vi "pxie_7962_fpga.vi"() -> ()   [LabVIEW 2014]
uses:
  <instrlib>/_niInstr/Streaming/v1/Common/Stream State.ctl
  FPGA_Controls/Init.ctl
  <vilib>/Platform/TimedLoop/XDataNode/timing_clust.ctl
  <vilib>/Platform/TimedLoop/XDataNode/nitl_modes.ctl
  <vilib>/Platform/TimedLoop/XDataNode/wakeup.ctl
  FPGA_Controls/Acquisition FIFOs Cluster.ctl
  <vilib>/rvi/Emulation/niFpgaSctlEmulationGetInTimedLoop.vi
  <vilib>/rvi/Emulation/niFpgaEmulationReportErrorSimple.vi
  <vilib>/rvi/Emulation/niFpgaGetClockAttributes.vi
  <vilib>/rvi/Emulation/niFpgaCriticalErrorInLSC.vi
  <vilib>/rvi/eio/common/nirviEmuTemplateMethod_errors.vi
  <instrlib>/_niInstr/Basic Elements/v1/FPGA/Private/Count Up U32.vi
  <vilib>/rvi/Memory/Memory_Emulation/niFpgaMemoryFastEmulationDramWriteAndRequestData.vi
  <vilib>/rvi/Memory/Memory_Emulation/niFpgaMemoryEmulationDramWriteAndRequestData.vi
  <vilib>/rvi/DataTransferAndStorage/Container/Common/niFpgaContainerGetUniqueNameForEmu.vi
  <vilib>/rvi/Memory/Memory_Emulation/niFpgaMemoryEmulationDramWriteAndRequestDataApplyByteEnables.vi
  <vilib>/rvi/interface/RandomDataEmulation/niFpgaRandomDataHandleErrors.vi
  <instrlib>/_niInstr/Basic Elements/v1/FPGA/Private/Count Up U64.vi
  <vilib>/rvi/DataTransferAndStorage/Container/Common/niFpgaContainerExecOnDevCompGetState.vi
  <vilib>/rvi/Emulation/niFpgaEmulationIsFPGAContextNoSignature.vi
  <vilib>/rvi/errors/niFpgaSetErrorForExecOnDevCompSimple.vi
  <vilib>/rvi/eio/common/nirviEmuReportErrorAndStop.vi
  <vilib>/rvi/FIFO/Fifo_Resource/nirvififoEmulationSetSize.vi
  <vilib>/rvi/FIFO/Fifo_Resource/nirviFifoEmulationQueueMgr.vi
  <instcachedir>/0/nirviFifoEmulationQueueMgr_E5CAEC123FF24DC58D834DCA3CDAA9B5.lvgen/nirviFifoEmulationQueueMgr_E5CAEC123FF24DC58D834DCA3CDAA9B5_003.vi
  <vilib>/rvi/FIFO/Fifo_Resource/nirvififoEmulationDetermineInputValidOut.vi
  <vilib>/rvi/FIFO/Fifo_Resource/nirvififoEmulationCreateLock.vi
  <vilib>/rvi/Emulation/niFpgaProcessEmulError.vi
  <vilib>/rvi/FIFO/Fifo_Resource/nirvififoEmulationObtainLock.vi
  <vilib>/rvi/FIFO/Fifo_Resource/nirvififoEmulationReleaseLock.vi
  <vilib>/rvi/occurrence/nirviWaitOnOccurrenceBase.vi
  <vilib>/rvi/errors/nirviReportUnexpectedCaseInternalError.vi
  <vilib>/rvi/errors/nirviReportUnexpectedCaseInternalError (U32).vi
  <vilib>/Utility/error.llb/Clear Errors.vi
  <vilib>/Platform/TimedLoop/XDataNode/XDataNode.xnode
  <vilib>/eio/EIONode/EIONode.xnode
  <vilib>/rvi/DataTransferAndStorage/Container/XNode/niFpgaContainer.xnode
  <vilib>/rvi/Memory/Memory_Emulation/niFpgaMemoryEmulationDramRetrieveData.vi
  <vilib>/rvi/interface/RandomDataEmulation/nirviRandomDataFpgaReadWriteTemplate.vi
  <vilib>/rvi/FIFO/Fifo_Resource/niFpgaFifoEmulationRefIn.vi
  <vilib>/Platform/TimedLoop/XDataNode/XDNodeRunTimeDep.lvlib
  <instrlib>/_niInstr/Streaming/v1/FPGA/niInstr Streaming v1 FPGA.lvlib
  <instrlib>/_niInstr/Basic Elements/v1/FPGA/niInstr Basic Elements v1 FPGA.lvlib
  <instrlib>/_niInstr/Streaming/v1/Common/niInstr Streaming v1 Common.lvlib
panel:
  in  "manual\ntrigger":bool
  out "Writes to DRAM":u64
  out "DRAM Write address":u32
  in  "Reset DRAM write address":bool
  in  "Reset DRAM read address":bool
  in  "trigger \ndelay":u64
  in  "Clear Trigger":bool
  in  "Output Debug Data":bool
  out "stream.metadata 0":u64
  in  "stream.request state 0":T1
  out "stream.samples transferred 0":u64
  out "stream.state 0":T1
  in  "stream.num samples 0":u64
  out "Writes to DMA":u64
  out "Samples Aquired":u64
  out "IO Module Init Done":bool
  in  "stream.num samples 1":u64
  out "stream.state 1":T1
  out "stream.samples transferred 1":u64
  in  "stream.request state 1":T1
  out "stream.metadata 1":u64
  # "Stream 0 (Aquisition Stream)"
  # "Throughput Diagnostics"
  # "Stream 1 (Transfer to Host Stream)"
  # "Settings & Resets"
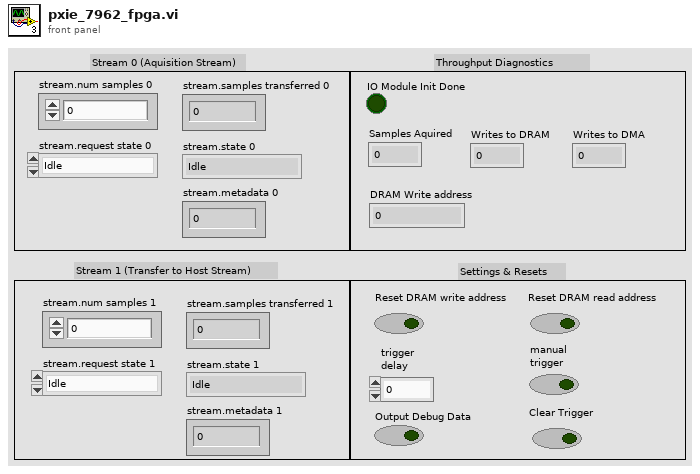
[diagram p1: front panel]
types:
  T1 = typedef "niInstr Streaming v1 Common.lvlib/Stream State.ctl" = enum8{"Idle", "Finite Transfer", "Continuous", "Done", "Error", "Not Ready", "Cancel"}
  T2 = typedef "Init.ctl" = enum16{"InitIOCheck", "ADCConfigForWrite", "SPIConfigWaitForSPIIdleFalse", "SPIConfigWaitForSPIIdleTrue", "ADCTurnOffInternalHighPassFilter", "SPIHighPassWaitForSPIIdleFalse", "SPIHighPassWaitForSPIIdleTrue"}
  T3 = typedef "XDNodeRunTimeDep.lvlib/timing_clust.ctl" = cluster{"Expected End [f-1]":u64, "Actual End [f-1]":u64, "Finished Late? [f-1]":bool, "Expected End [i-1]":u64, "Actual End [i-1]":u64, "Finished Late? [i-1]":bool, "Expected Start [i]":u64, "Actual Start [i]":u64, "Expected Start [f]":u64, "Actual Start [f]":u64, "Source Name":string, "Structure Name":string, "Period":i64, "Deadline":i64, "Offset":i64, "Start":i64, "Priority":i32, "Timeout":i32, "Mode":T4, "Wakeup Reason":T5, "Error":errorcluster, "Source Type":string, "Secondary Source Type":string, "Global End Time":u64, "Global Start Time":u64, "Frame Duration":u64, "Iteration Duration":u64, "Assigned CPU":i32, "I/O Scan Engine Mode":u32}
  T4 = typedef "XDNodeRunTimeDep.lvlib/nitl_modes.ctl" = enum32{"No Change", "Process missed periods, maintain original phase", "Discard missed periods, maintain original phase", "Process missed periods, ignore original phase", "Discard missed periods, ignore original phase"}
  T5 = typedef "XDNodeRunTimeDep.lvlib/wakeup.ctl" = enum32{"Normal", "Aborted", "Asynchronous wakeup", "Timing source error", "Timed loop error", "Timeout"}
  T6 = typedef "Acquisition FIFOs Cluster.ctl" = cluster{"FIFO 0":refnum<k21>, "FIFO 1":refnum<k21>, "FIFO 2":refnum<k21>, "FIFO 3":refnum<k21>, "FIFO 4":refnum<k21>, "FIFO 5":refnum<k21>, "FIFO 6":refnum<k21>, "FIFO 7":refnum<k21>}
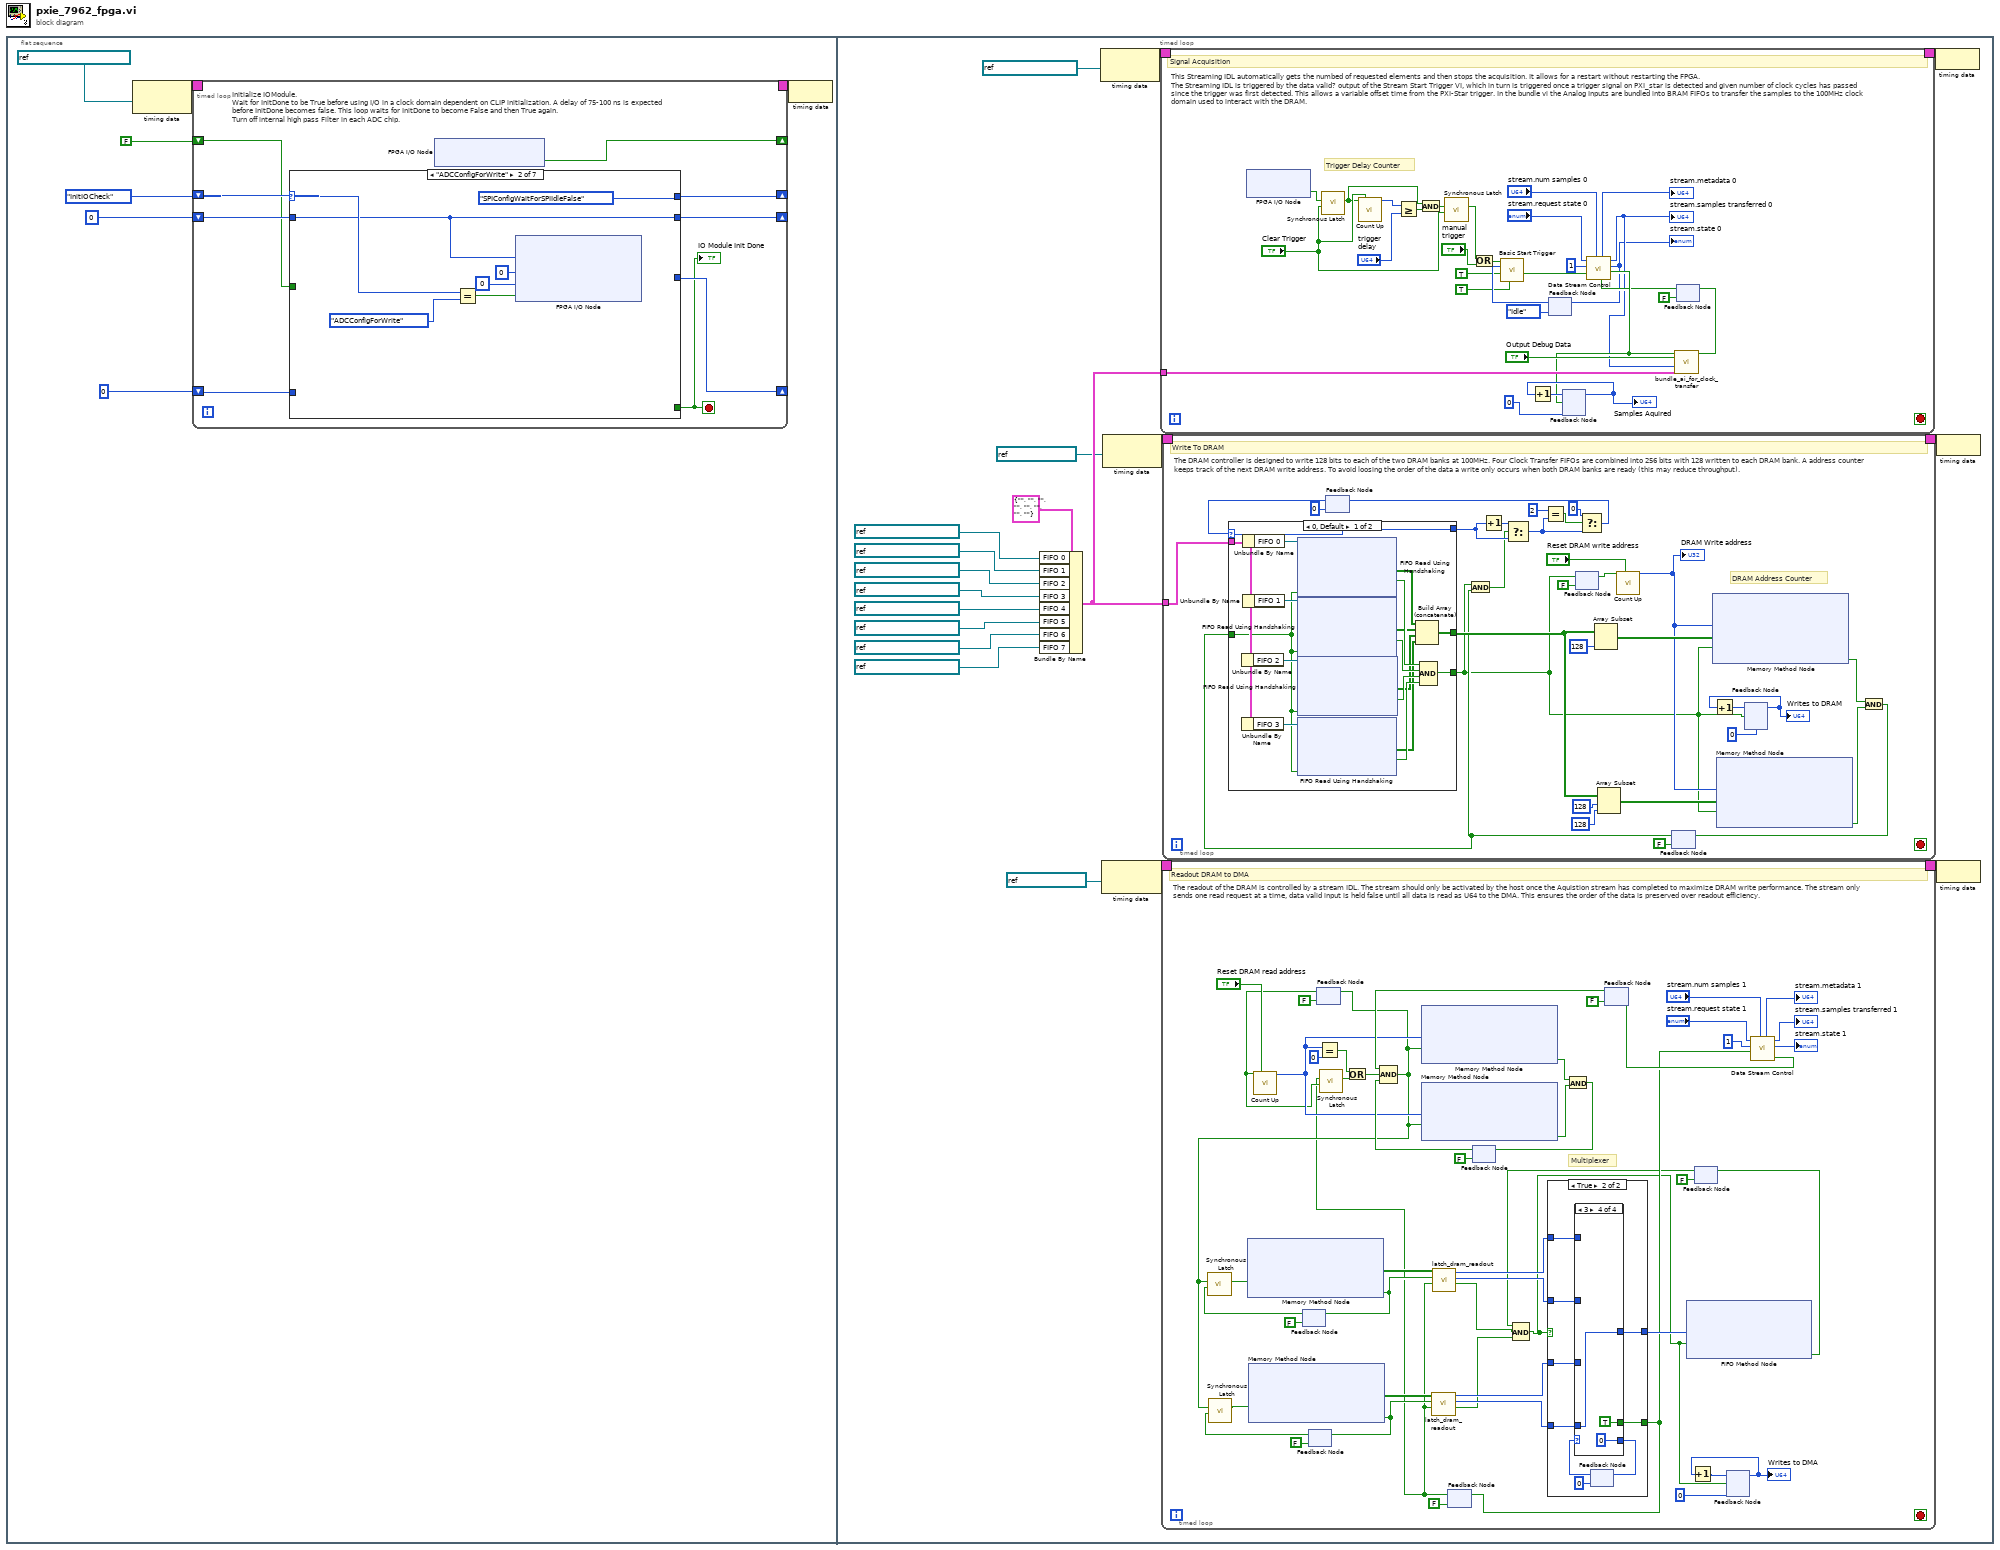
[diagram p0: block diagram]
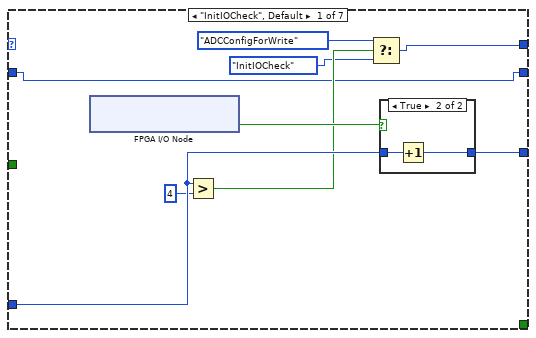
[diagram p2: hidden frame]
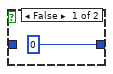
[diagram p3: hidden frame]
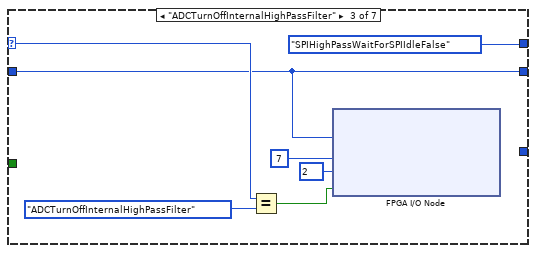
[diagram p4: hidden frame]
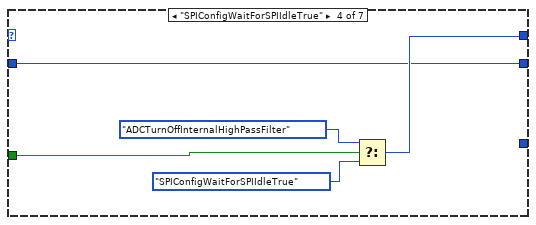
[diagram p5: hidden frame]
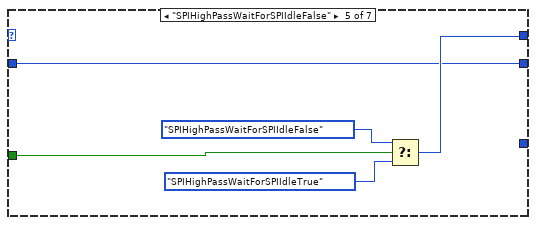
[diagram p6: hidden frame]
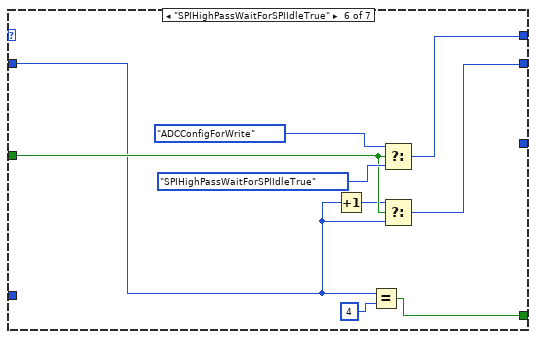
[diagram p7: hidden frame]
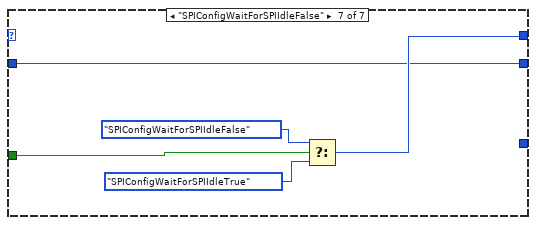
[diagram p8: hidden frame]
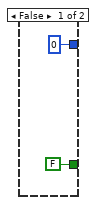
[diagram p9: hidden frame]
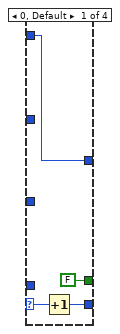
[diagram p10: hidden frame]
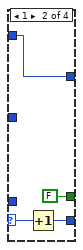
[diagram p11: hidden frame]
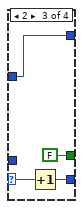
[diagram p12: hidden frame]
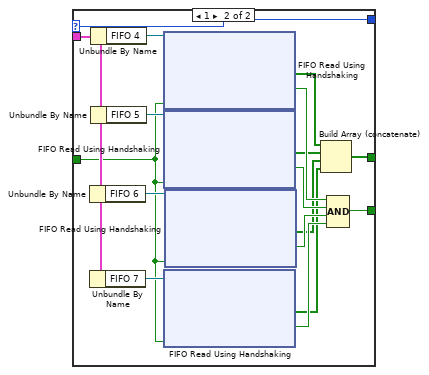
[diagram p13: hidden frame]
diagram:
  n1 = flat-sequence {
    frame #0 {
      # "Initialize IOModule.\nWait for InitDone to be True before using I/O in a clock domain dependent on CLIP initialization. A delay of 75-100 ns is expected before InitDone becomes false. This loop waits for InitDone to become False and then True again.\nTurn off internal high pass Filter in each ADC chip."
      n2 = node-c288(refnum<k21> "40 MHz Onboard Clock" ("Source Name")) -> (w7:T3)
      n3 = timed-loop {
        shift-right: [w16] -> _
        shift-left: u16 0 -> [w15]
        timing: w7 -> [_]
        timing-out: [_] -> w6
        shift-right: [w14] -> _
        shift-left: Init."InitIOCheck" -> [w13]
        shift-right: [w11] -> _
        shift-left: u8 0 -> [w12]
        shift-right: [w10] -> _
        shift-left: FALSE ("IO Module\\cSpiIdle") -> [w9]
        stop <- w8 stop-if-true
        n4 = case shown="\"ADCConfigForWrite\"" w13 {
          selector: w13 -> [_ w32 w39 _ _ _ _]
          tunnel: [w25 _ _ _ _ _ _] -> w16
          tunnel: w15 -> [w24 _ _ _ _ _ _]
          tunnel: [w21 Init."SPIConfigWaitForSPIIdleFalse" Init."SPIHighPassWaitForSPIIdleFalse" ("y") w44 w50 w59 w63] -> w14
          tunnel: [_ _ _ _ _ w57 _] -> w8
          tunnel: w12 -> [w17 w30 w37 w43 w48 w54 w62]
          tunnel: [w17 w30 w37 w43 w48 w53 w62] -> w11
          tunnel: w9 -> [_ _ _ w45 w49 w56 w66]
          frame "InitIOCheck", Default {
            n5 = xnode "FPGA I/O Node"() -> ("IO Module\\InitDone"=w22:bool)  [unwired: 1 in, 1 out]
            n6 = Greater?(x=w24, y=u16 4) -> (0:w20:bool)
            n7 = Select(t=Init."ADCConfigForWrite", s=w20, f=Init."InitIOCheck") -> (s? t:f=w21:T2)
            n8 = case shown="True" w22 {
              tunnel: [u16 0 w28] -> w25
              tunnel: w24 -> [_ w27]
              frame False {
              }
              frame True {
                n9 = Increment(x=w27) -> (x+1=w28:u16)
              }
            }
          }
          frame "ADCConfigForWrite" {
            n10 = Equal?(x=w32, y=Init."ADCConfigForWrite") -> (x = y?=w33:bool)
            n11 = xnode "FPGA I/O Node"("IO Module\\cSpiDevice"=w30, "IO Module\\cSpiAddr"=u16 0 ("IO Module\\cSpiAddr"), "IO Module\\cSpiWrData"=u16 0 ("IO Module\\cSpiWrData"), "IO Module\\cSpiWriteEn"=w33) -> ()  [unwired: 4 in, 4 out]
          }
          frame "ADCTurnOffInternalHighPassFilter" {
            n12 = Equal?(x=w39, y=Init."ADCTurnOffInternalHighPassFilter") -> (x = y?=w40:bool)
            n13 = xnode "FPGA I/O Node"("IO Module\\cSpiDevice"=w37, "IO Module\\cSpiAddr"=u16 7 ("IO Module\\cSpiAddr"), "IO Module\\cSpiWrData"=u16 2 ("IO Module\\cSpiWrData"), "IO Module\\cSpiWriteEn"=w40) -> ()  [unwired: 4 in, 4 out]
          }
          frame "SPIConfigWaitForSPIIdleTrue" {
            n14 = Select(t=Init."ADCTurnOffInternalHighPassFilter", s=w45, f=Init."SPIConfigWaitForSPIIdleTrue") -> (s? t:f=w44:T2)
          }
          frame "SPIHighPassWaitForSPIIdleFalse" {
            n15 = Select(t=Init."SPIHighPassWaitForSPIIdleFalse", s=w49, f=Init."SPIHighPassWaitForSPIIdleTrue") -> (s? t:f=w50:T2)
          }
          frame "SPIHighPassWaitForSPIIdleTrue" {
            n16 = Increment(x=w54) -> (x+1=w55:u8)
            n17 = Equal?(x=w54, y=u8 4) -> (x = y?=w57:bool)
            n18 = Select(t=Init."ADCConfigForWrite", s=w56, f=Init."SPIHighPassWaitForSPIIdleTrue") -> (s? t:f=w59:T2)
            n19 = Select(t=w55, s=w56, f=w54) -> (s? t:f=w53:u8)
          }
          frame "SPIConfigWaitForSPIIdleFalse" {
            n20 = Select(t=Init."SPIConfigWaitForSPIIdleFalse", s=w66, f=Init."SPIConfigWaitForSPIIdleTrue") -> (s? t:f=w63:T2)
          }
        }
        "IO Module Init Done" <- w8
        n21 = xnode "FPGA I/O Node"() -> ("IO Module\\cSpiIdle"=w10:bool)  [unwired: 1 in, 1 out]
      }
      n22 = node-c288(w6) -> ()
    }
    frame #1 {
      n23 = Bundle By Name(cluster=T6 {"FIFO 0"="", "FIFO 1"="", "FIFO 2"="", "FIFO 3"="", "FIFO 4"="", "FIFO 5"="", "FIFO 6"="", "FIFO 7"=""} ("FIFO Refs"), "FIFO 0"=refnum<k21> "Clock Transfer FIFO 0" ("FIFO In"), "FIFO 1"=refnum<k21> "Clock Transfer FIFO 1" ("FIFO In"), "FIFO 2"=refnum<k21> "Clock Transfer FIFO 2" ("FIFO In"), "FIFO 3"=refnum<k21> "Clock Transfer FIFO 3" ("FIFO In"), "FIFO 4"=refnum<k21> "Clock Transfer FIFO 4" ("FIFO In"), "FIFO 5"=refnum<k21> "Clock Transfer FIFO 5" ("FIFO In"), "FIFO 6"=refnum<k21> "Clock Transfer FIFO 6" ("FIFO In"), "FIFO 7"=refnum<k21> "Clock Transfer FIFO 7" ("FIFO In")) -> (w76:T6)
      n24 = node-c288(refnum<k21> "IO Module Clock 0" ("Source Name")) -> (w91:T3)
      n25 = node-c288(refnum<k21> "100 MHz Clock" ("Source Name")) -> (w87:T3)
      n26 = node-c288(refnum<k21> "100 MHz Clock" ("Source Name")) -> (w89:T3)
      n27 = timed-loop {
        timing: w91 -> [_]
        timing-out: [_] -> w90
        tunnel: w76 -> [w268]
        stop <- _ stop-if-true
        # "Trigger Delay Counter"
        # "This Streaming IDL automatically gets the numbed of requested elements and then stops the acquisition. It allows for a restart without restarting the FPGA. \nThe Streaming IDL is triggered by the data valid? output of the Stream Start Trigger VI, which in turn is triggered once a trigger signal on PXI_star is detected and given number of clock cycles has passed since the trigger was first detected. This allows a variable offset time from the PXI-Star trigger. In the bundle vi the Analog Inputs are bundled into BRAM FIFOs to transfer the samples to the 100MHz clock domain used to interact with the DRAM."
        # "Signal Acquisition"
        n28 = xnode "FPGA I/O Node"() -> ("PXI_Star"=w254:bool)  [unwired: 1 in, 1 out]
        n29 = call <instrlib>:"Synchronous Latch.vi"("clear"="Clear Trigger", "set"=w254) -> ("out"=w248:bool)  [unwired: 9 in]
        n30 = call-poly <instrlib>:"Count Up.vi"("increment"=w248, "reset"="Clear Trigger") -> ("count out"=w253:u64)  [unwired: 13 in]
        n31 = Greater Or Equal?(x=w253, y="trigger \ndelay") -> (x >= y?=w249:bool)
        n32 = And(x=w248, y=w249) -> (x .and. y?=w247:bool)
        n33 = call <instrlib>:"Synchronous Latch.vi"("clear"="Clear Trigger", "set"=w247) -> ("out"=w246:bool)  [unwired: 9 in]
        n34 = Or(x=w246, y="manual\ntrigger") -> (x .or. y?=w244:bool)
        n35 = feedback #1(Stream_State."Idle" ("stream.state 0")) -> (w258:T1)
        n36 = call <instrlib>:"Basic Start Trigger.vi"("ready for start trigger"=TRUE, "data valid?"=TRUE, "stream.state"=w258, "start trigger"=w244) -> ("data valid"=w251:bool)  [unwired: 7 in]
        n37 = feedback #2(u64 0) -> (w269:u64)
        "Samples Aquired" <- w269
        n38 = Increment(x=w269) -> (x+1=w270:u64)
        n39 = feedback #3(FALSE ("Ready for Input")) -> (w265:bool)
        n40 = call <instrlib>:"Data Stream Control.vi"("ready for input?"=w265, "stream.num samples 0"="stream.num samples 0", "data valid"=w251, "element count"=u16 1, "stream.request state 0"="stream.request state 0") -> ("send data"=w266:bool, "stream.state 0"=w262:T1, "stream.samples transferred 0"=w263:u64, "stream.metadata 0"=→"stream.metadata 0":u64)  [unwired: 2 in, 1 out]
        "stream.state 0" <- w262
        "stream.samples transferred 0" <- w263
        n41 = feedback-in #1(w262) -> ()
        n42 = feedback-in #2(w270, w266) -> ()
        n43 = call "bundle_ai_for_clock_transfer.vi"("FIFO Refs"=w268, "sample"=w263, "Debug"="Output Debug Data", "Input Valid"=w266) -> ("Ready for Input"=w273:bool)  [unwired: 7 in]
        n44 = feedback-in #3(w273) -> ()
      }
      n45 = timed-loop {
        timing: w87 -> [_]
        timing-out: [_] -> w86
        stop <- _ stop-if-true
        # "Multiplexer"
        # "The readout of the DRAM is controlled by a stream IDL. The stream should only be activated by the host once the Aquistion stream has completed to maximize DRAM write performance. The stream only sends one read request at a time, data valid input is held false until all data is read as U64 to the DMA. This ensures the order of the data is preserved over readout efficiency."
        # "Readout DRAM to DMA"
        n46 = feedback #4(FALSE ("Output Valid")) -> (w106:bool)
        n47 = feedback #5(FALSE ("Output Valid")) -> (w103:bool)
        n48 = feedback #6(FALSE) -> (w113:bool)
        n49 = call-poly <instrlib>:"Count Up.vi"("increment"=w113, "reset"="Reset DRAM read address") -> ("count out"=w118:u32)  [unwired: 13 in]
        n50 = Equal?(x=w118, y=u32 0) -> (x = y?=w115:bool)
        n51 = feedback #7(FALSE) -> (w99:bool)
        n52 = call <instrlib>:"Synchronous Latch.vi"("clear"=w113, "set"=w99) -> ("out"=w114:bool)  [unwired: 9 in]
        n53 = Or(x=w115, y=w114) -> (x .or. y?=w116:bool)
        n54 = feedback #8(FALSE) -> (w120:bool)
        n55 = feedback #9(FALSE ("request data")) -> (w119:bool)
        n56 = Compound Arithmetic op=AND(w119, w116, w120) -> (w102:bool)
        n57 = call <instrlib>:"Synchronous Latch.vi"("clear"=w106, "set"=w102) -> ("out"=w109:bool)  [unwired: 9 in]
        n58 = call <instrlib>:"Synchronous Latch.vi"("clear"=w103, "set"=w102) -> ("out"=w108:bool)  [unwired: 9 in]
        n59 = xnode ("Memory Method Node")("Ready for Output"=w109) -> ("Data"=w132:bool[], "Output Valid"=w107:bool)  [unwired: 1 in, 1 out]
        n60 = xnode ("Memory Method Node")("Ready for Output"=w108) -> ("Data"=w101:bool[], "Output Valid"=w100:bool)  [unwired: 1 in, 1 out]
        n61 = feedback-in #4(w107) -> ()
        n62 = feedback-in #5(w100) -> ()
        n63 = feedback-in #6(w102) -> ()
        n64 = xnode ("Memory Method Node")("Address"=w118, "Input Valid"=w102) -> ("Ready for Input"=w124:bool)  [unwired: 1 in, 1 out]
        n65 = xnode ("Memory Method Node")("Address"=w118, "Input Valid"=w102) -> ("Ready for Input"=w123:bool)  [unwired: 1 in, 1 out]
        n66 = call "latch_dram_readout.vi"("Reset"=w99, "Output Valid"=w100, "Data"=w101) -> ("Lateched Output Valid"=w92:bool, "latched U64 1"=w97:u64, "lateched U64 0"=w98:u64)  [unwired: 6 in]
        n67 = call "latch_dram_readout.vi"("Reset"=w99, "Output Valid"=w107, "Data"=w132) -> ("Lateched Output Valid"=w93:bool, "latched U64 1"=w131:u64, "lateched U64 0"=w130:u64)  [unwired: 6 in]
        n68 = And(x=w124, y=w123) -> (x .and. y?=w122:bool)
        n69 = feedback-in #8(w122) -> ()
        n70 = feedback #10(FALSE ("Ready for Input")) -> (w94:bool)
        n71 = Compound Arithmetic op=AND(w94, w93, w92) -> (w95:bool)
        n72 = case shown="True" w95 {
          tunnel: w97 -> [_ w152]
          tunnel: w98 -> [_ w151]
          tunnel: w131 -> [_ w150]
          tunnel: w130 -> [_ w149]
          tunnel: [u64 0 ("q") w145] -> w128
          tunnel: [FALSE w144] -> w112
          frame False {
          }
          frame True {
            n73 = feedback #11(i16 0) -> (w146:i16)
            n74 = case shown="3" w146 {
              selector: w146 -> [w155 w159 w163 _]
              tunnel: w152 -> [_ _ _ w166]
              tunnel: w151 -> [_ _ w162 _]
              tunnel: w150 -> [_ w158 _ _]
              tunnel: w149 -> [w154 _ _ _]
              tunnel: [w156 w160 w164 i16 0] -> w148
              tunnel: [w154 w158 w162 w166] -> w145
              tunnel: [FALSE FALSE FALSE TRUE] -> w144
              frame 0, Default {
                n75 = Increment(x=w155) -> (x+1=w156:i16)
              }
              frame 1 {
                n76 = Increment(x=w159) -> (x+1=w160:i16)
              }
              frame 2 {
                n77 = Increment(x=w163) -> (x+1=w164:i16)
              }
              frame 3 {
              }
            }
            n78 = feedback-in #11(w148) -> ()
          }
        }
        n79 = feedback-in #7(w112) -> ()
        n80 = xnode ("FIFO Method Node")("Element"=w128, "Input Valid"=w95) -> ("Ready for Input"=w129:bool)  [unwired: 1 in, 1 out]
        n81 = feedback-in #10(w129) -> ()
        n82 = feedback #12(u64 0) -> (w135:u64)
        "Writes to DMA" <- w135
        n83 = Increment(x=w135) -> (x+1=w136:u64)
        n84 = feedback-in #12(w136, w95) -> ()
        n85 = call <instrlib>:"Data Stream Control.vi"("stream.num samples 0"="stream.num samples 1", "data valid"=w112, "element count"=u16 1, "stream.request state 0"="stream.request state 1") -> ("request data"=w126:bool, "stream.state 0"=→"stream.state 1":T1, "stream.samples transferred 0"=→"stream.samples transferred 1":u64, "stream.metadata 0"=→"stream.metadata 1":u64)  [unwired: 3 in, 1 out]
        n86 = feedback-in #9(w126) -> ()
      }
      n87 = timed-loop {
        timing: w89 -> [_]
        timing-out: [_] -> w88
        tunnel: w76 -> [w203]
        stop <- _ stop-if-true
        # "DRAM Address Counter"
        # "The DRAM controller is designed to write 128 bits to each of the two DRAM banks at 100MHz. Four Clock Transfer FIFOs are combined into 256 bits with 128 written to each DRAM bank. A address counter keeps track of the next DRAM write address. To avoid loosing the order of the data a write only occurs when both DRAM banks are ready (this may reduce throughput)."
        # "Write To DRAM"
        n88 = feedback #13(i16 0 ("t")) -> (w202:i16)
        n89 = feedback #14(FALSE ("Output Valid")) -> (w183:bool)
        n90 = call-poly <instrlib>:"Count Up.vi"("increment"=w183, "reset"="Reset DRAM write address") -> ("count out"=w182:u32)  [unwired: 13 in]
        "DRAM Write address" <- w182
        n91 = feedback #15(FALSE) -> (w175:bool)
        n92 = case shown="0, Default" w202 {
          selector: w202 -> [w219 w236]
          tunnel: w203 -> [w205 w222]
          tunnel: [w217 w234] -> w180
          tunnel: [w210 w227] -> w174
          tunnel: [w219 w236] -> w200
          tunnel: w175 -> [w204 w221]
          frame 0, Default {
            n93 = Unbundle By Name(w205) -> ("FIFO 2"=w216:refnum<k21>)
            n94 = Unbundle By Name(w205) -> ("FIFO 3"=w215:refnum<k21>)
            n95 = Unbundle By Name(w205) -> ("FIFO 0"=w220:refnum<k21>)
            n96 = Unbundle By Name(w205) -> ("FIFO 1"=w218:refnum<k21>)
            n97 = xnode ("FIFO Read Using Handshaking")("Ready for Output"=w204, "FIFO In"=w220) -> ("Element"=w209:bool[], "Output Valid"=w214:bool)  [unwired: 1 out]
            n98 = xnode ("FIFO Read Using Handshaking")("Ready for Output"=w204, "FIFO In"=w218) -> ("Element"=w208:bool[], "Output Valid"=w213:bool)  [unwired: 1 out]
            n99 = xnode ("FIFO Read Using Handshaking")("Ready for Output"=w204, "FIFO In"=w215) -> ("Element"=w206:bool[], "Output Valid"=w211:bool)  [unwired: 1 out]
            n100 = xnode ("FIFO Read Using Handshaking")("Ready for Output"=w204, "FIFO In"=w216) -> ("Element"=w207:bool[], "Output Valid"=w212:bool)  [unwired: 1 out]
            n101 = Build Array (concatenate)(w209, w208, w207, w206) -> (w217:bool[])
            n102 = Compound Arithmetic op=AND(w214, w213, w212, w211) -> (w210:bool)
          }
          frame 1 {
            n103 = Unbundle By Name(w222) -> ("FIFO 6"=w233:refnum<k21>)
            n104 = Unbundle By Name(w222) -> ("FIFO 7"=w232:refnum<k21>)
            n105 = Unbundle By Name(w222) -> ("FIFO 4"=w237:refnum<k21>)
            n106 = Unbundle By Name(w222) -> ("FIFO 5"=w235:refnum<k21>)
            n107 = xnode ("FIFO Read Using Handshaking")("Ready for Output"=w221, "FIFO In"=w237) -> ("Element"=w226:bool[], "Output Valid"=w231:bool)  [unwired: 1 out]
            n108 = xnode ("FIFO Read Using Handshaking")("Ready for Output"=w221, "FIFO In"=w235) -> ("Element"=w225:bool[], "Output Valid"=w230:bool)  [unwired: 1 out]
            n109 = xnode ("FIFO Read Using Handshaking")("Ready for Output"=w221, "FIFO In"=w232) -> ("Element"=w223:bool[], "Output Valid"=w228:bool)  [unwired: 1 out]
            n110 = xnode ("FIFO Read Using Handshaking")("Ready for Output"=w221, "FIFO In"=w233) -> ("Element"=w224:bool[], "Output Valid"=w229:bool)  [unwired: 1 out]
            n111 = Build Array (concatenate)(w226, w225, w224, w223) -> (w234:bool[])
            n112 = Compound Arithmetic op=AND(w231, w230, w229, w228) -> (w227:bool)
          }
        }
        n113 = And(x=w174, y=w175) -> (x .and. y?=w176:bool)
        n114 = Increment(x=w200) -> (x+1=w201:i16)
        n115 = Select(t=w201, s=w176, f=w200) -> (s? t:f=w198:i16)
        n116 = Equal?(x=i16 2, y=w198) -> (x = y?=w197:bool)
        n117 = feedback-in #14(w174) -> ()
        n118 = Select(t=i16 0, s=w197, f=w198) -> (s? t:f=w196:i16)
        n119 = feedback-in #13(w196) -> ()
        n120 = Array Subset(array=w180, length=128) -> (w189:bool[])  [unwired: 1 in]
        n121 = Array Subset(array=w180, index=128, length=128) -> (w188:bool[])
        n122 = xnode ("Memory Method Node")("Address"=w182, "Data"=w189, "Input Valid"=w174) -> ("Ready for Input"=w186:bool)  [unwired: 1 in, 1 out]
        n123 = xnode ("Memory Method Node")("Address"=w182, "Data"=w188, "Input Valid"=w174) -> ("Ready for Input"=w187:bool)  [unwired: 1 in, 1 out]
        n124 = feedback #16(u64 0) -> (w178:u64)
        "Writes to DRAM" <- w178
        n125 = Increment(x=w178) -> (x+1=w179:u64)
        n126 = feedback-in #16(w179, w174) -> ()
        n127 = And(x=w186, y=w187) -> (x .and. y?=w185:bool)
        n128 = feedback-in #15(w185) -> ()
      }
      n129 = node-c288(w90) -> ()
      n130 = node-c288(w88) -> ()
      n131 = node-c288(w86) -> ()
    }
  }
